vi "10.1 Writing and reading Data to a file.vi"() -> ()   [LabVIEW 2019]
uses:
  <vilib>/DAQmx/read.llb/DAQmx Read (Analog 2D DBL NChan NSamp).vi
  <vilib>/DAQmx/create/channels.llb/DAQmx Create Channel (AI-Voltage-Basic).vi
  <vilib>/DAQmx/configure/timing.llb/DAQmx Timing (Sample Clock).vi
  <vilib>/DAQmx/miscellaneous.llb/DAQmx Fill In Error Info.vi
  <vilib>/Utility/file.llb/Write Delimited Spreadsheet (string).vi
  <vilib>/Utility/file.llb/Write Delimited Spreadsheet (DBL).vi
  <resource>/objmgr/daqmx.rc
panel:
  in  "File Path Control":path
  out "Waveform Graph":dbl[][](graph)
  out "Actual Sample Rate (Hz)":dbl
  in  "Configuration Control":T1={"number of samples"=-1, "Minimum Value"=-1.0, "Maximum Value"=-1.0, "physical channels"="Multi_I-O/ai0", "Desired Sample Rate (Hz)"=-1.0, "sample mode"=10178} {"sample mode" items=["Finite Samples"=10178, "Continuous Samples"=10123, "Hardware Timed Single Point"=12522]}
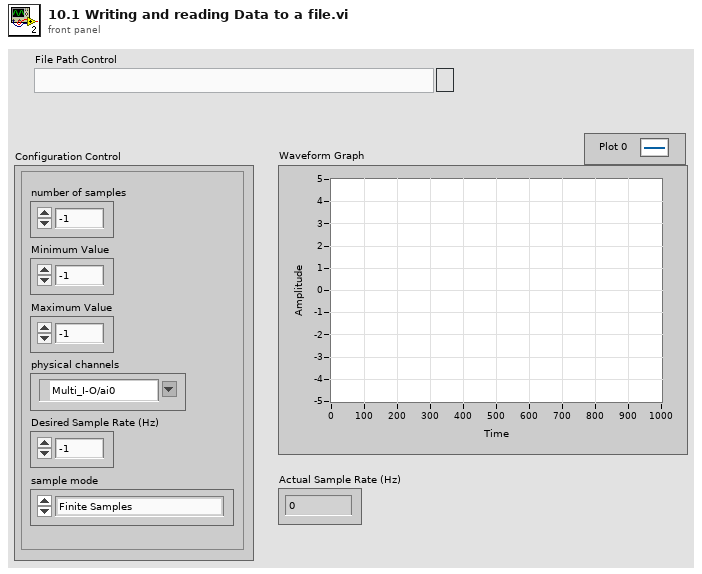
[diagram p1: front panel]
types:
  T1 = cluster{"number of samples":i32, "Minimum Value":dbl, "Maximum Value":dbl, "physical channels":tag, "Desired Sample Rate (Hz)":dbl, "sample mode":i32}
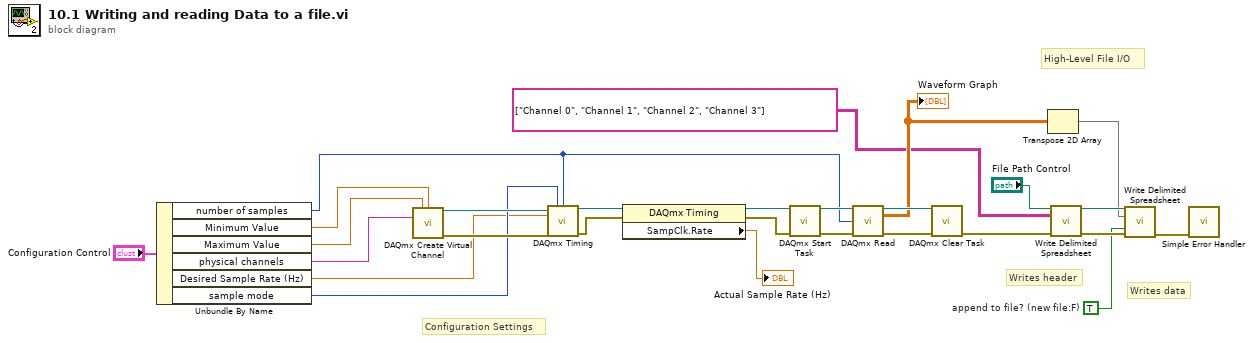
[diagram p0: block diagram]
diagram:
  w3 = TRUE  # append to file? (new file:F)
  # "Writes data"
  # "Writes header"
  # "Configuration Settings"
  # "High-Level File I/O"
  n1 = Unbundle By Name("Configuration Control") -> ("number of samples"=w10:i32, "Minimum Value"=w23:dbl, "Maximum Value"=w24:dbl, "physical channels"=w22:tag, "Desired Sample Rate (Hz)"=w20:dbl, "sample mode"=w21:i32)
  n2 = call-poly <vilib>:"DAQmx Create Virtual Channel.vi"("maximum value"=w24, "minimum value"=w23, "physical channels"=w22) -> ("task out"=w27:refnum<k21>, "error out"=w26:errorcluster)  [unwired: 11 in]
  n3 = call-poly <vilib>:"DAQmx Timing.vi"("task/channels in"=w27, "sample mode"=w21, "samples per channel"=w10, "rate"=w20, "error in"=w26) -> ("task out"=w18:refnum<k21>, "error out"=w19:errorcluster)  [unwired: 9 in]
  n4 = property class="DAQmx Timing"(reference=w18, error in=w19) -> (reference out=w14:refnum<k21>, error out=w13:errorcluster, "SampClk.Rate"=→"Actual Sample Rate (Hz)":dbl)
  n5 = call <vilib>:"DAQmx Start Task.vi"("task/channels in"=w14, "error in"=w13) -> ("task out"=w16:refnum<k21>, "error out"=w12:errorcluster)  [unwired: 12 in]
  n6 = call-poly <vilib>:"DAQmx Read.vi"("task/channels in"=w16, "number of samples per channel"=w10, "error in"=w12) -> ("task out"=w15:refnum<k21>, "data"=w5:dbl[][], "error out"=w11:errorcluster)  [unwired: 10 in]
  "Waveform Graph" <- w5
  n7 = call <vilib>:"DAQmx Clear Task.vi"("task in"=w15, "error in"=w11) -> ("error out"=w6:errorcluster)  [unwired: 13 in]
  n8 = Transpose 2D Array(2D array=w5) -> (transposed array=w4:dbl[][])
  n9 = call-poly <vilib>:"Write Delimited Spreadsheet.vi"("file path (dialog if empty)"="File Path Control", "2D data"=string[][] [["Channel 0", "Channel 1", "Channel 2", "Channel 3"]], "error in (no error)"=w6) -> ("new file path (Not A Path if cancelled)"=w8:path, "error out"=w7:errorcluster)  [unwired: 11 in]
  n10 = call-poly <vilib>:"Write Delimited Spreadsheet.vi"("file path (dialog if empty)"=w8, "2D data"=w4, "append to file? (new file:F)"=w3, "error in (no error)"=w7) -> ("error out"=w2:errorcluster)  [unwired: 10 in, 1 out]
  n11 = call <vilib>:"Simple Error Handler.vi"("error in (no error)"=w2) -> ()  [unwired: 4 in, 5 out]
